vi "sv_ConcatenateArrayIndicies.vi"(7 "indices":i32[](array[numeric])) -> (6 "subset lengths":i32[](array[numeric]), 10 "subset start indices":i32[](array[numeric]))   [LabVIEW 2017]
doc: "This VI converts a list of ascending array indices into a set of array subsets. The two output arrays are the start indices and lengths, respectively, of the subsets. Compacting the array of indices into a smaller set of array subsets can reduce the amount of times the delete from array VI needs to be called."
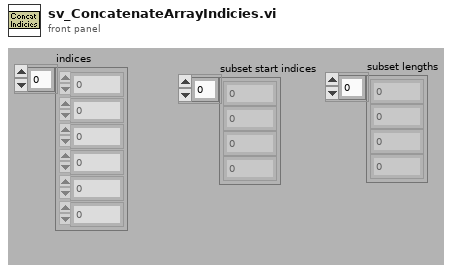
[diagram p1: front panel]
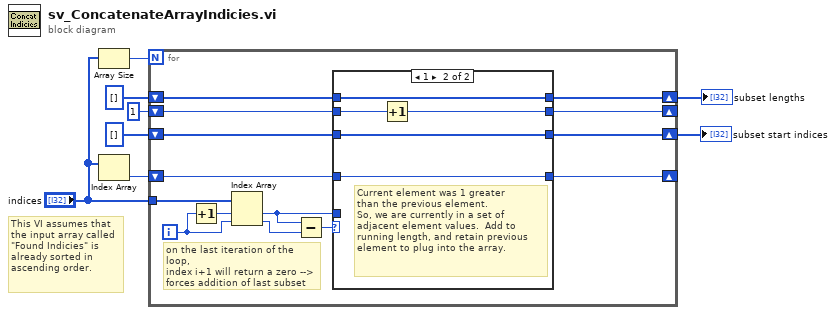
[diagram p0: block diagram]
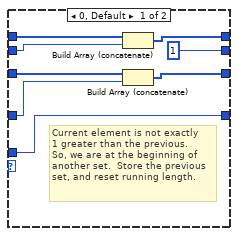
[diagram p2: hidden frame]
diagram:
  # "This VI assumes that\nthe input array called\n\"Found Indicies\" is\nalready sorted in\nascending order."
  n1 = Array Size(array="indices") -> (size(s)=w2:i32)
  n2 = Index Array(array="indices") -> (element=w4:i32)  [unwired: 1 in]
  n3 = for {
    N: w2 -> [_]
    shift-right: [w21] -> w8
    shift-left: i32[] [] ("Found Indicies") -> [w22]
    shift-right: [w19] -> w7
    shift-left: i32[] [] ("Found Indicies") -> [w20]
    shift-right: [w17] -> _
    shift-left: 1 -> [w18]
    shift-right: [w16] -> _
    shift-left: w4 -> [w15]
    tunnel: "indices" -> [w13]
    i -> [w9]
    # "on the last iteration of the loop,\nindex i+1 will return a zero --> forces addition of last subset"
    n4 = Increment(x=w9) -> (x+1=w14:i32)
    n5 = Index Array(array=w13, index #1=w14, index #2=w9) -> (element #1=w12:i32, element #2=w11:i32)
    n6 = Subtract(x=w12, y=w11) -> (x-y=w10:i32)
    n7 = case shown="1" w10 {
      tunnel: w22 -> [w30 w32]
      tunnel: w15 -> [w29 w31]
      tunnel: [w28 w32] -> w21
      tunnel: w20 -> [w27 w33]
      tunnel: [w26 w33] -> w19
      tunnel: w18 -> [w25 w35]
      tunnel: [1 w34] -> w17
      tunnel: [w23 w31] -> w16
      tunnel: w12 -> [w23 _]
      frame 0, Default {
        # "Current element is not exactly\n1 greater than the previous.\nSo, we are at the beginning of\nanother set.  Store the previous\nset, and reset running length."
        n8 = Build Array (concatenate)(w27, w25) -> (w26:i32[])
        n9 = Build Array (concatenate)(w30, w29) -> (w28:i32[])
      }
      frame 1 {
        # "Current element was 1 greater\nthan the previous element.\nSo, we are currently in a set of\nadjacent element values.  Add to \nrunning length, and retain previous \nelement to plug into the array."
        n10 = Increment(x=w35) -> (x+1=w34:i32)
      }
    }
  }
  "subset start indices" <- w8
  "subset lengths" <- w7
